vi "Configure Measurement (Burst Power).vi"(0 "VISA resource name":refnum<visa-resource-name>, 1 "Measurement Method (0: Above Threshold Level)":u16(ring) items=["Above Threshold Level", "Measured  Burst Width"], 2 "Enable Auto Measured Burst Width (T: Enable)":bool=TRUE, 3 "Measured Burst Width (0.000542.77 s)":dbl=0.00054277 format="%#.8g", 5 "Average Type (1: RMS)":u16(ring)=1 items=["Log", "RMS"], 7 "Threshold Type (0: Absolute)":u16(ring) items=["Absolute", "Relative"], 9 "Threshold Level (-30 dB)":dbl=-30.0 format="%#.6g", 11 "error in (no error)":errorcluster) -> (4 "VISA resource name out":refnum<visa-resource-name>, 15 "error out":errorcluster)   [LabVIEW 2014, in "Agilent ESA PSA Series.lvlib"]
doc: "Sets up the burst power measurement."
uses:
  Agilent ESA PSA Series.lvlib
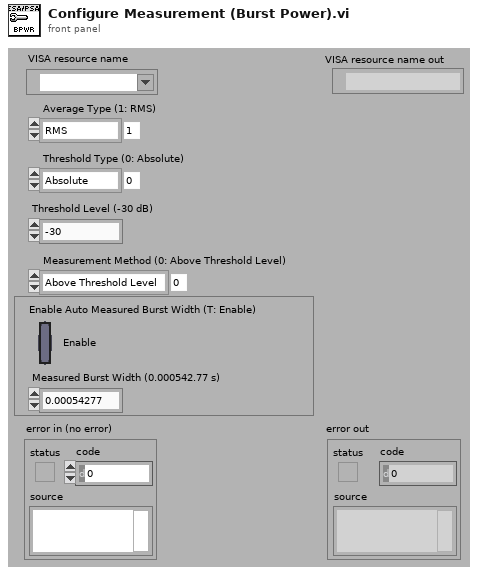
[diagram p1: front panel]
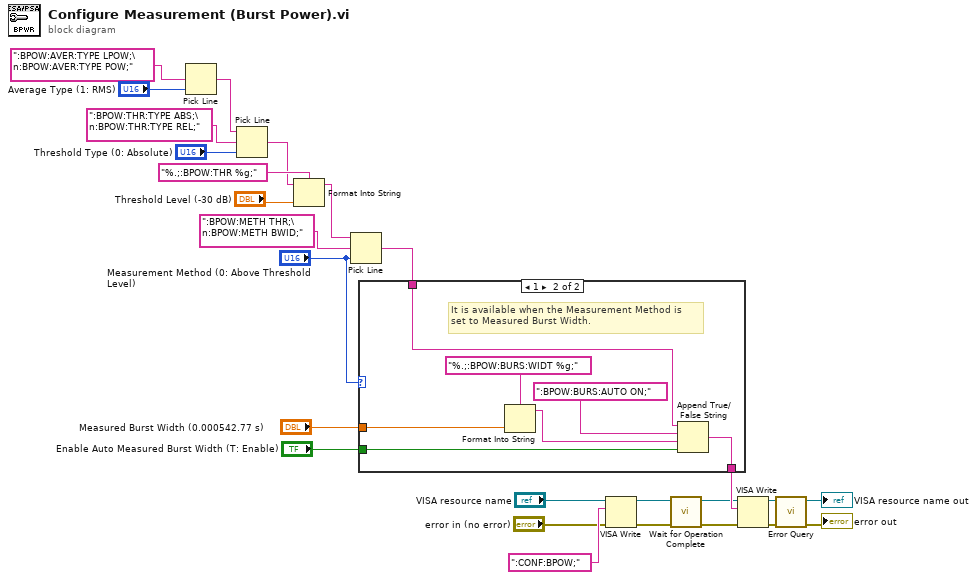
[diagram p0: block diagram]
diagram:
  n1 = Pick Line(multi-line string=":BPOW:AVER:TYPE LPOW;\n:BPOW:AVER:TYPE POW;" ("string (\"\")"), line index="Average Type (1: RMS)") -> (output string=w16:string)  [unwired: 1 in]
  n2 = Pick Line(string ("")=w16, multi-line string=":BPOW:THR:TYPE ABS;\n:BPOW:THR:TYPE REL;" ("string (\"\")"), line index="Threshold Type (0: Absolute)") -> (output string=w17:string)
  n3 = Format Into String(format string="%.;:BPOW:THR %g;", initial string=w17, "Threshold Level (-30 dB)") -> (resulting string=w15:string)  [unwired: 1 in, 1 out]
  n4 = Pick Line(string ("")=w15, multi-line string=":BPOW:METH THR;\n:BPOW:METH BWID;" ("string (\"\")"), line index="Measurement Method (0: Above Threshold Level)") -> (output string=w11:string)
  n5 = case shown="1" "Measurement Method (0: Above Threshold Level)" {
    tunnel: "Enable Auto Measured Burst Width (T: Enable)" -> [_ w32]
    tunnel: "Measured Burst Width (0.000542.77 s)" -> [_ w31]
    tunnel: w11 -> [w27 w29]
    tunnel: [w27 w28] -> w10
    frame 0, Default {
    }
    frame 1 {
      # "It is available when the Measurement Method is\nset to Measured Burst Width."
      n6 = Format Into String(format string="%.;:BPOW:BURS:WIDT %g;", w31) -> (resulting string=w34:string)  [unwired: 2 in, 1 out]
      n7 = Append True/False String(1:w32, 2:w34, 3:":BPOW:BURS:AUTO ON;" ("true string"), 4:w29) -> (0:w28:string)
    }
  }
  n8 = VISA Write(VISA resource name="VISA resource name", write buffer=":CONF:BPOW;" ("string (\"\")"), error in (no error)="error in (no error)") -> (VISA resource name out=w4:refnum<visa-resource-name>, error out=w3:errorcluster)  [unwired: 1 out]
  n9 = call "Wait for Operation Complete.vi"("error in (no error)"=w3, "VISA resource name"=w4) -> ("error out"=w2:errorcluster, "VISA resource name out"=w1:refnum<visa-resource-name>)  [unwired: 8 in]
  n10 = VISA Write(VISA resource name=w1, write buffer=w10, error in (no error)=w2) -> (VISA resource name out=w8:refnum<visa-resource-name>, error out=w7:errorcluster)  [unwired: 1 out]
  n11 = call "Error Query.vi"("error in (no error)"=w7, "VISA resource name"=w8) -> ("error out"=→"error out":errorcluster, "VISA resource name out"=→"VISA resource name out":refnum<visa-resource-name>)  [unwired: 6 in, 2 out]
